vi "Compiled Get Node Frames.vi"(6 "Type":T3, 8 "error in (no error)":errorcluster, 9 "Refs in":T2 {"Trigger Refs" format="%.0x"; "Disable Refs" format="%.0x"; "VS Refs" format="%.0x"}, 10 "Database in":refnum<k21>, 11 "Section Ref in":T1 format="%.0x") -> (0 "error out":errorcluster, 1 "Refs out":T2 {"Trigger Refs" format="%.0x"; "Disable Refs" format="%.0x"; "VS Refs" format="%.0x"}, 2 "Counter and Protection Frames":T1[](array[typedef]) format="%.0x", 3 "Standard Frames":T4[](array[typedef]))   [LabVIEW 2015, in "J1939 Addon System Explorer.lvlib"]
uses:
  J1939 Addon System Explorer.lvlib
  <vilib>/NI Veristand/Custom Device API/Custom Device Item Ref.ctl
  Shared/Types/Outgoing Frame Settings.ctl
  Shared/Types/Outgoing Event Trigger Types.ctl
  Shared/Types/Exported Frame Type.ctl
  Types/Compiled Refs.ctl
  Shared/J1939 Utilities/SubVIs/Convert CAN Arb ID to J1939 ID.vi
  Shared/SubVIs/Constants.vi
  <vilib>/NI VeriStand/Custom Device API/Custom Device API.lvlib
  Shared/J1939 Addon Shared.lvlib
  Shared/J1939 Utilities/J1939 Utilities.lvlib
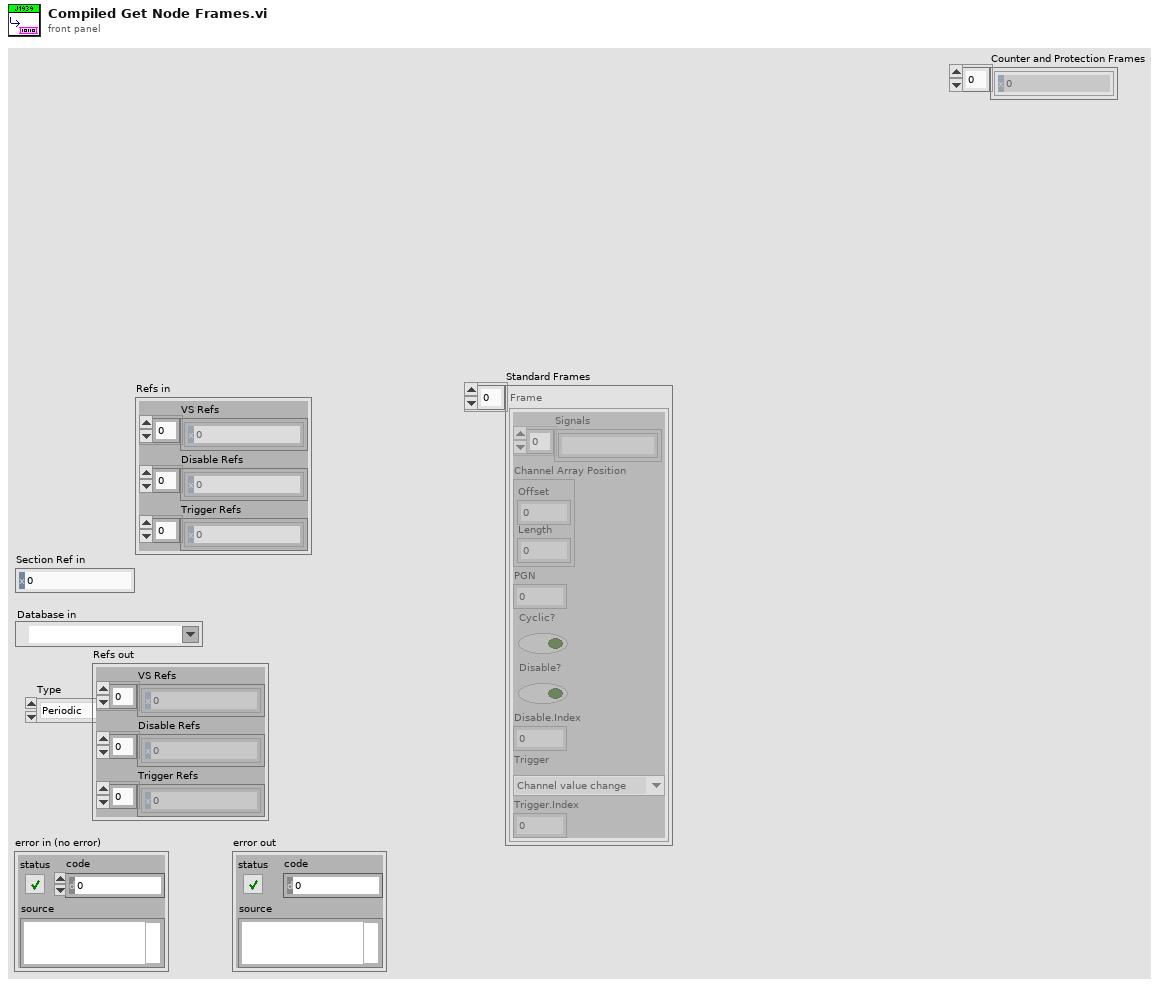
[diagram p1: front panel]
types:
  T1 = typedef "Custom Device API.lvlib/Custom Device Item Ref.ctl" = u64
  T2 = typedef "J1939 Addon System Explorer.lvlib/Compiled Refs.ctl" = cluster{"VS Refs":T1[], "Disable Refs":T1[], "Trigger Refs":T1[]}
  T3 = typedef "J1939 Addon Shared.lvlib/Exported Frame Type.ctl" = enum16{"Periodic", "Event", "Periodic/Event"}
  T4 = typedef "J1939 Addon Shared.lvlib/Outgoing Frame Settings.ctl" = cluster{"Signals":string[], "Channel Array Position":cluster{"Offset":u32, "Length":u32}, "PGN":u32, "Cyclic?":bool, "Disable?":bool, "Disable.Index":i32, "Trigger":T5, "Trigger.Index":i32}
  T5 = typedef "J1939 Addon Shared.lvlib/Outgoing Event Trigger Types.ctl" = enum16{"Channel value change", "Trigger channel (not zero)", "Channel value change or trigger channel (not zero)", "Trigger channel (any value change)", "Channel value change or trigger channel (any value change)"}
  T6 = typedef "Custom Device API.lvlib/Custom Device Item Info.ctl" = cluster{"Name":string, "Is Channel":bool, "GUID":string, "Is Waveform":bool}
  T7 = typedef "J1939 Addon Shared.lvlib/Frame.Settings.ctl" = cluster{"ID":u32, "Disable Transmission":bool, "Disable Transmission Ref":T1, "Transmit Trigger":T5, "Transmit Trigger Ref":T1}
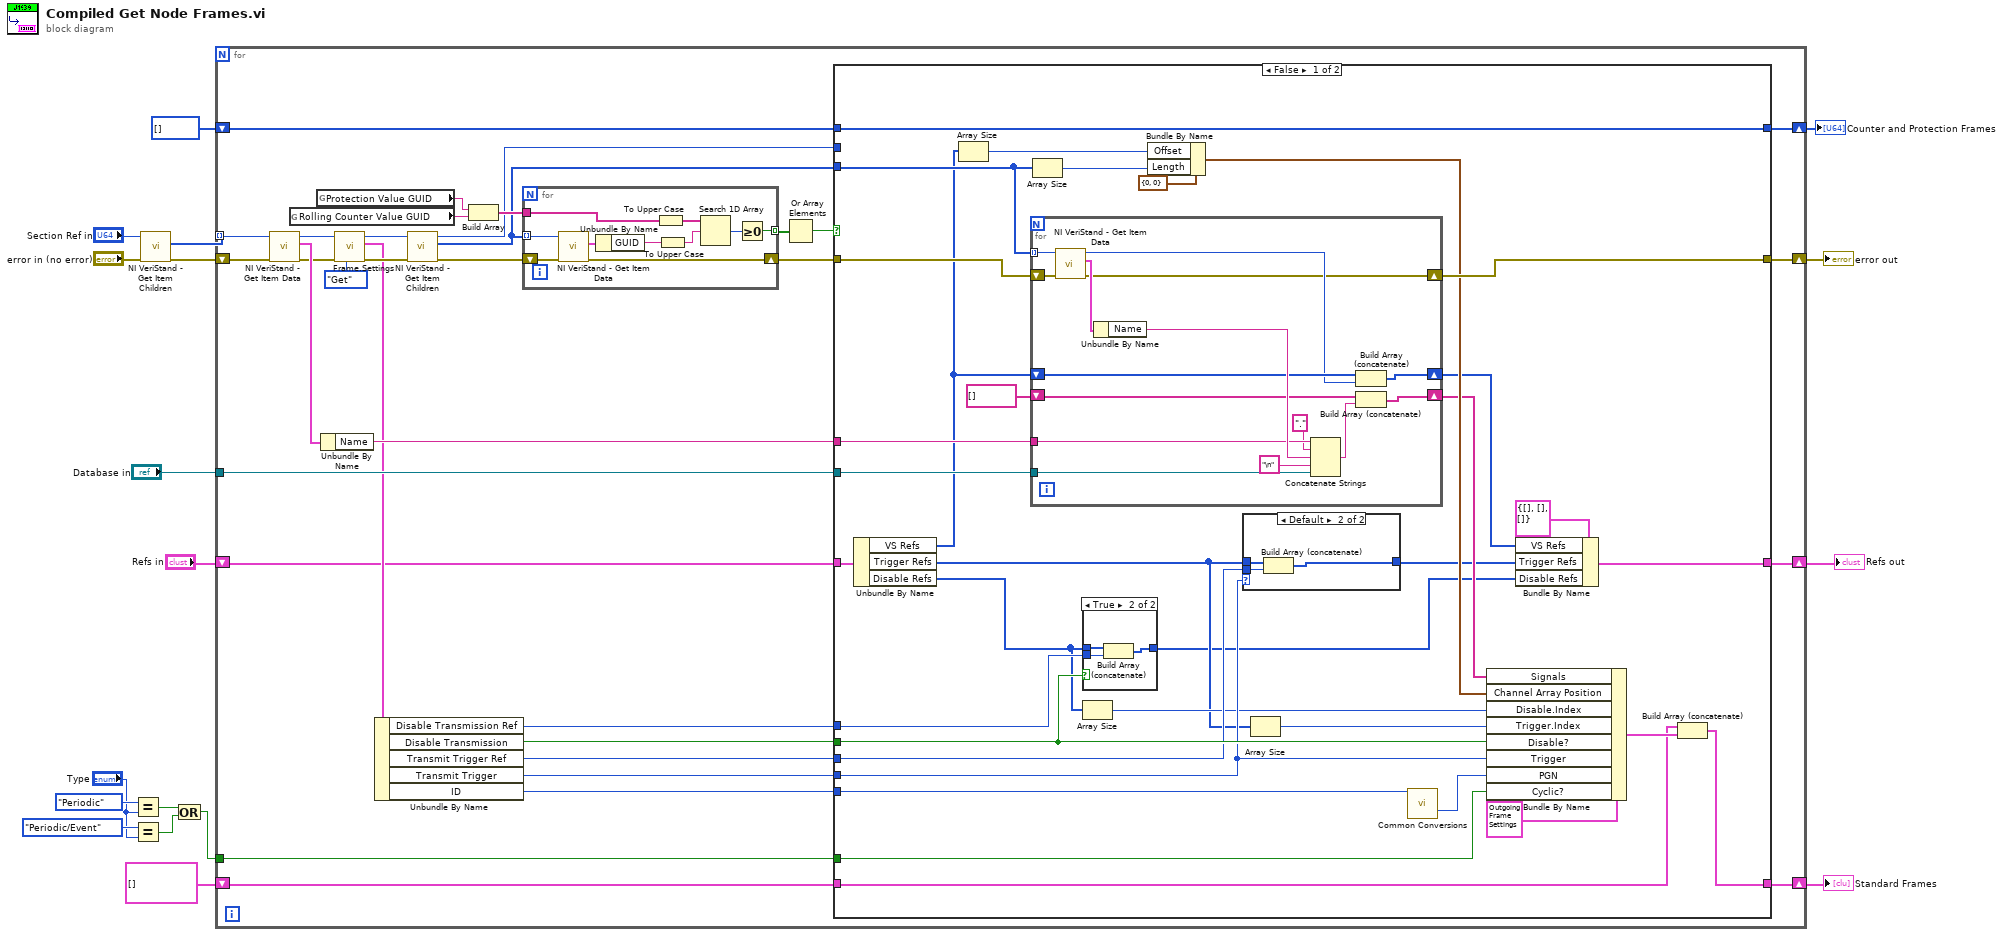
[diagram p0: block diagram]
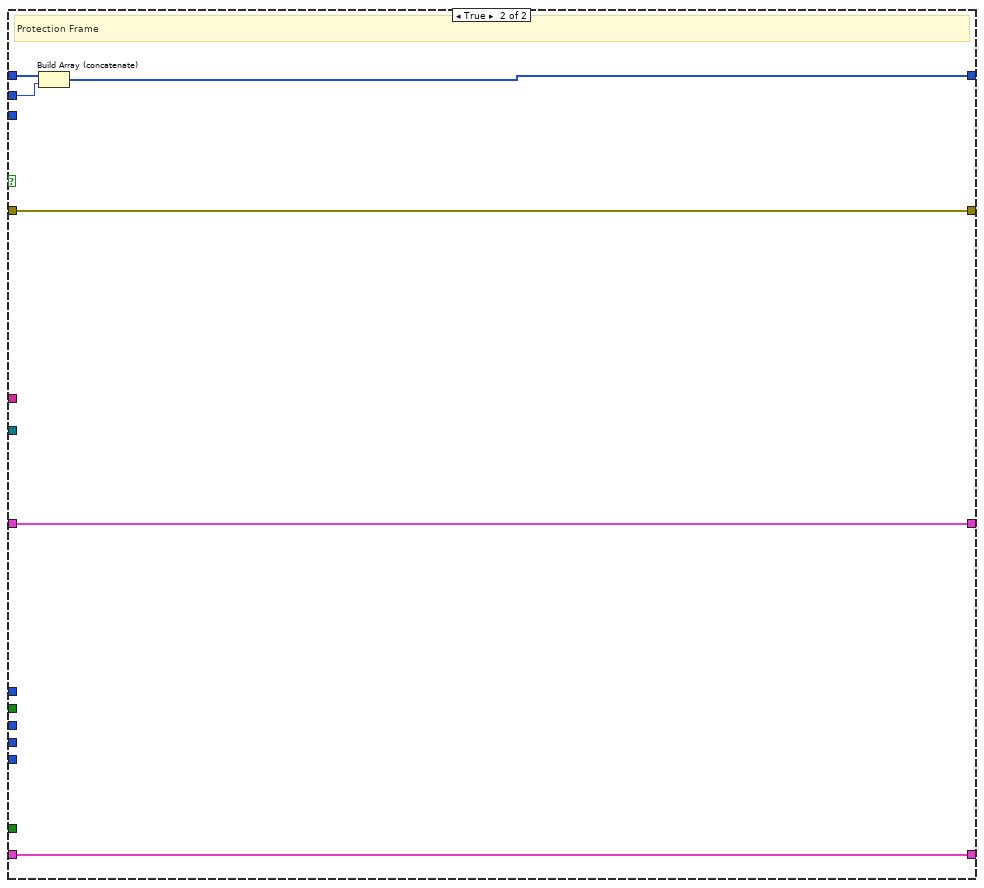
[diagram p4: hidden frame]
diagram:
  n1 = Equal?(x=Exported_Frame_Type."Periodic", y="Type") -> (x = y?=w6:bool)
  n2 = Equal?(x=Exported_Frame_Type."Periodic/Event", y="Type") -> (x = y?=w5:bool)
  n3 = call <vilib>:"NI VeriStand - Get Item Children.vi"("error in (no error)"="error in (no error)", "Item Ref in"="Section Ref in") -> ("error out"=w15:errorcluster, "Child Refs"=w17:T1[])  [unwired: 6 in, 2 out]
  n4 = Compound Arithmetic op=OR(w6, w5) -> (w3:bool)
  n5 = for {
    shift-right: [w43] -> w18
    shift-left: w15 -> [w48]
    tunnel: w17 -> [w49] mode=indexing
    tunnel: "Database in" -> [w42]
    tunnel: w3 -> [w41]
    shift-right: [w23] -> w11
    shift-left: "Refs in" -> [w24]
    shift-right: [w21] -> w9
    shift-left: T4[] [] -> [w22]
    shift-right: [w20] -> w1
    shift-left: T1[] [] -> [w19]
    n6 = call <vilib>:"NI VeriStand - Get Item Data.vi"("error in (no error)"=w48, "Item Ref in"=w49) -> ("error out"=w45:errorcluster, "Item Info"=w47:T6, "Item Ref out"=w46:T1)  [unwired: 6 in, 1 out]
    n7 = global read "Constants.vi" "Rolling Counter Value GUID"() -> (w33:string)
    n8 = global read "Constants.vi" "Protection Value GUID"() -> (w32:string)
    n9 = Unbundle By Name(w47) -> ("Name"=w44:string)
    n10 = call "Frame.Settings.vi"("Action"=enum8{"Get", "Set"}."Get", "error in (no error)"=w45, "Item Ref in"=w46) -> ("error out"=w51:errorcluster, "Frame.Settings"=w39:T7, "Item Ref out"=w50:T1)  [unwired: 6 in]
    n11 = Unbundle By Name(w39) -> ("Disable Transmission Ref"=w36:T1, "Disable Transmission"=w37:bool, "Transmit Trigger Ref"=w35:T1, "Transmit Trigger"=w34:T5, "ID"=w38:u32)
    n12 = call <vilib>:"NI VeriStand - Get Item Children.vi"("error in (no error)"=w51, "Item Ref in"=w50) -> ("error out"=w29:errorcluster, "Child Refs"=w27:T1[], "Item Ref out"=w25:T1)  [unwired: 6 in, 1 out]
    n13 = Build Array(w32, w33) -> (w31:string[])
    n14 = for {
      tunnel: w27 -> [w122] mode=indexing
      tunnel: w31 -> [w120]
      tunnel: [w116] -> w30 mode=indexing
      shift-right: [w115] -> w28
      shift-left: w29 -> [w123]
      n15 = call <vilib>:"NI VeriStand - Get Item Data.vi"("error in (no error)"=w123, "Item Ref in"=w122) -> ("error out"=w115:errorcluster, "Item Info"=w124:T6)  [unwired: 6 in, 2 out]
      n16 = Unbundle By Name(w124) -> ("GUID"=w121:string)
      n17 = To Upper Case(1:w120) -> (0:w119:string[])
      n18 = To Upper Case(1:w121) -> (0:w118:string)
      n19 = Search 1D Array(1D array=w119, element=w118) -> (index of element=w117:i32)  [unwired: 1 in]
      n20 = Greater Or Equal To 0?(x=w117) -> (x >= 0?=w116:bool)
    }
    n21 = Or Array Elements(Boolean array=w30) -> (logical OR=w26:bool)
    n22 = case shown="False" w26 {
      tunnel: w44 -> [w83 _]
      tunnel: [w82 w114] -> w43
      tunnel: w42 -> [w81 _]
      tunnel: w41 -> [w77 _]
      tunnel: w38 -> [w74 _]
      tunnel: w37 -> [w73 _]
      tunnel: w36 -> [w72 _]
      tunnel: w35 -> [w71 _]
      tunnel: w34 -> [w70 _]
      tunnel: w28 -> [w67 w114]
      tunnel: w27 -> [w66 _]
      tunnel: w25 -> [_ w110]
      tunnel: w24 -> [w64 w113]
      tunnel: [w56 w113] -> w23
      tunnel: w22 -> [w54 w112]
      tunnel: [w53 w112] -> w21
      tunnel: [w52 w109] -> w20
      tunnel: w19 -> [w52 w111]
      frame False {
        n23 = Unbundle By Name(w64) -> ("VS Refs"=w61:T1[], "Trigger Refs"=w62:T1[], "Disable Refs"=w63:T1[])
        n24 = Array Size(array=w61) -> (size(s)=w65:i32)
        n25 = for {
          shift-right: [w97] -> w82
          shift-left: w67 -> [w107]
          tunnel: w66 -> [w108] mode=indexing
          shift-right: [w102] -> w59
          shift-left: w61 -> [w103]
          tunnel: w83 -> [w101]
          tunnel: w81 -> [w99]
          shift-right: [w104] -> w75
          shift-left: string[] [] ("Signals") -> [w98]
          n26 = call <vilib>:"NI VeriStand - Get Item Data.vi"("error in (no error)"=w107, "Item Ref in"=w108) -> ("error out"=w97:errorcluster, "Item Info"=w106:T6, "Item Ref out"=w100:T1)  [unwired: 6 in, 1 out]
          n27 = Unbundle By Name(w106) -> ("Name"=w105:string)
          n28 = Concatenate Strings(w101, "." ("string"), w105, "\n" ("string"), w99) -> (w94:string)
          n29 = Build Array (concatenate)(w103, w100) -> (w102:T1[])
          n30 = Build Array (concatenate)(w98, w94) -> (w104:string[])
        }
        n31 = Array Size(array=w66) -> (size(s)=w84:i32)
        n32 = case shown="True" w73 {
          tunnel: w63 -> [w90 w93]
          tunnel: w72 -> [_ w92]
          tunnel: [w90 w91] -> w57
          frame False {
          }
          frame True {
            n33 = Build Array (concatenate)(w93, w92) -> (w91:T1[])
          }
        }
        n34 = Array Size(array=w63) -> (size(s)=w68:i32)
        n35 = Bundle By Name(cluster=cluster{"Offset":u32, "Length":u32} {"Offset"=0, "Length"=0} ("Channel Array Position"), "Offset"=w65, "Length"=w84) -> (w80:cluster{"Offset":u32, "Length":u32})
        n36 = case shown="Default" w70 {
          tunnel: w62 -> [w86 w89]
          tunnel: w71 -> [_ w88]
          tunnel: [w86 w87] -> w58
          frame "Channel value change" {
          }
          frame Default {
            n37 = Build Array (concatenate)(w89, w88) -> (w87:T1[])
          }
        }
        n38 = Array Size(array=w62) -> (size(s)=w69:i32)
        n39 = call-poly "Common Conversions.vi"("Arb ID"=w74) -> ("PGN"=w78:u32)  [unwired: 11 in, 3 out]
        n40 = Bundle By Name(cluster=T4 {"Signals"=[], "Channel Array Position"={"Offset"=0, "Length"=0}, "PGN"=0, "Cyclic?"=FALSE, "Disable?"=FALSE, "Disable.Index"=0, "Trigger"=enum."Channel value change", "Trigger.Index"=0} ("Frame"), "Signals"=w75, "Channel Array Position"=w80, "Disable.Index"=w68, "Trigger.Index"=w69, "Disable?"=w73, "Trigger"=w70, "PGN"=w78, "Cyclic?"=w77) -> (w55:T4)
        n41 = Bundle By Name(cluster=T2 {"VS Refs"=[], "Disable Refs"=[], "Trigger Refs"=[]} ("Refs in"), "VS Refs"=w59, "Trigger Refs"=w58, "Disable Refs"=w57) -> (w56:T2)
        n42 = Build Array (concatenate)(w54, w55) -> (w53:T4[])
      }
      frame True {
        # "Protection Frame"
        n43 = Build Array (concatenate)(w111, w110) -> (w109:T1[])
      }
    }
  }
  "error out" <- w18
  "Standard Frames" <- w9
  "Refs out" <- w11
  "Counter and Protection Frames" <- w1
